vi "Console_Merge.vi"(5 "New Lines":refnum<vi>, 6 "Buffer Size":i32=-1, 7 "Console":refnum<vi>, 9 "Text read":string, 11 "Console In":string) -> (3 "Console Out":string)   [LabVIEW 2022 SP3]
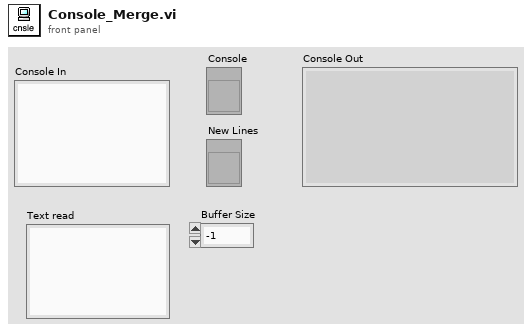
[diagram p1: front panel]
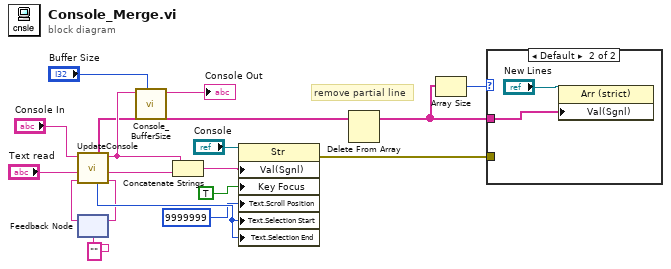
[diagram p0: block diagram]
diagram:
  # "remove partial line"
  n1 = feedback #1("" ("Left over raw")) -> (w5:string)
  n2 = call "UpdateConsole.vi"("from last time raw"=w5, "New Text"="Text read", "Console"="Console In") -> ("Left over raw"=w7:string, "left over fixed"=w10:string, "Console Out"=w17:string, "cursor out"=w15:i32, "lines"=w2:string[])  [unwired: 3 in, 1 out]
  n3 = feedback-in #1(w7) -> ()
  n4 = call "Console_BufferSize.vi"("Buffer Size"="Buffer Size", "Console Out in"=w17) -> ("Console Out out"=→"Console Out":string)  [unwired: 9 in]
  n5 = Concatenate Strings(w17, w10) -> (w14:string)
  n6 = property on="Property Node" class="Str"(reference="Console", "Val(Sgnl)"=w14, "Key Focus"=TRUE, "Text.Scroll Position"=u32 9999999, "Text.Selection Start"=w15, "Text.Selection End"=w15) -> (error out=w3:errorcluster)  [unwired: 1 in, 1 out]
  n7 = Delete From Array(array=w2) -> (array with subset deleted=w1:string[])  [unwired: 2 in, 1 out]
  n8 = Array Size(array=w1) -> (size(s)=w4:i32)
  n9 = case shown="Default" w4 {
    tunnel: w3 -> [_ _]
    tunnel: w1 -> [_ w19]
    frame 0 {
    }
    frame Default {
      n10 = property on="Property Node" class="Arr (strict)"(reference="New Lines", "Val(Sgnl)"=w19) -> ()  [unwired: 1 in, 2 out]
    }
  }
